vi "delay chart.vi"(8 "Spec":dbl, 9 "Des.":string="TDD11", 10 "Impedance Data":dbl[](array[numeric]), 11 "Time Array":dbl[](array[numeric])) -> (0 "Test Summary":string, 1 "test passed?":bool=TRUE caption="Test Pass?", 2 "Test Data":T2, 3 "Impedance Chart":T1(graph), 5 "delay":dbl)   [LabVIEW 2011]
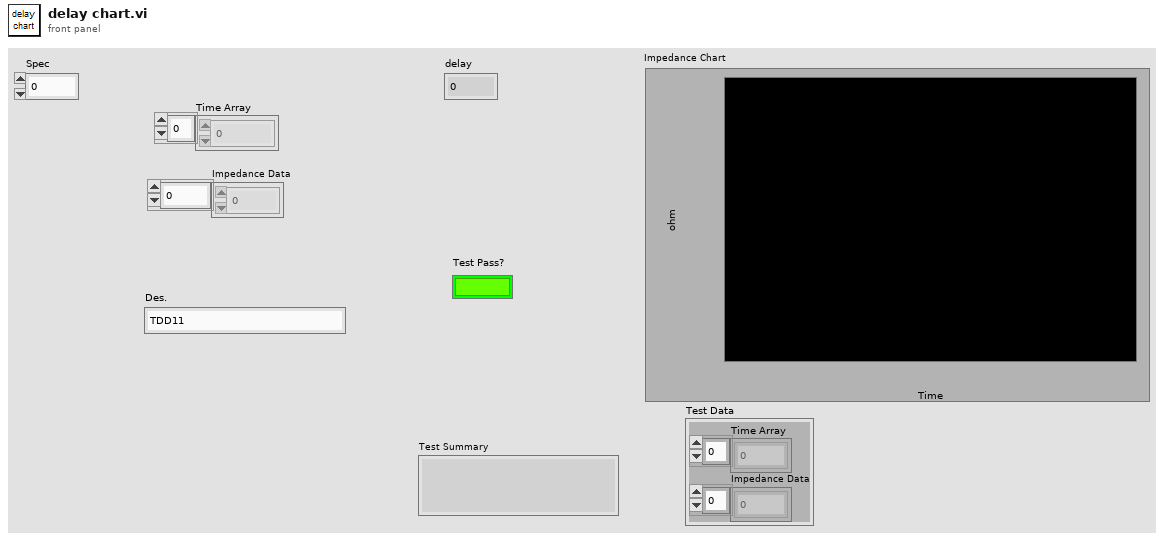
[diagram p1: front panel]
types:
  T1 = cluster{"Time Array":dbl[], "Lower Spec":dbl[]}[]
  T2 = cluster{"Time Array":dbl[], "Impedance Data":dbl[]}
  T3 = cluster{"Time Array":dbl[], "Impedance Data":dbl[]}[]
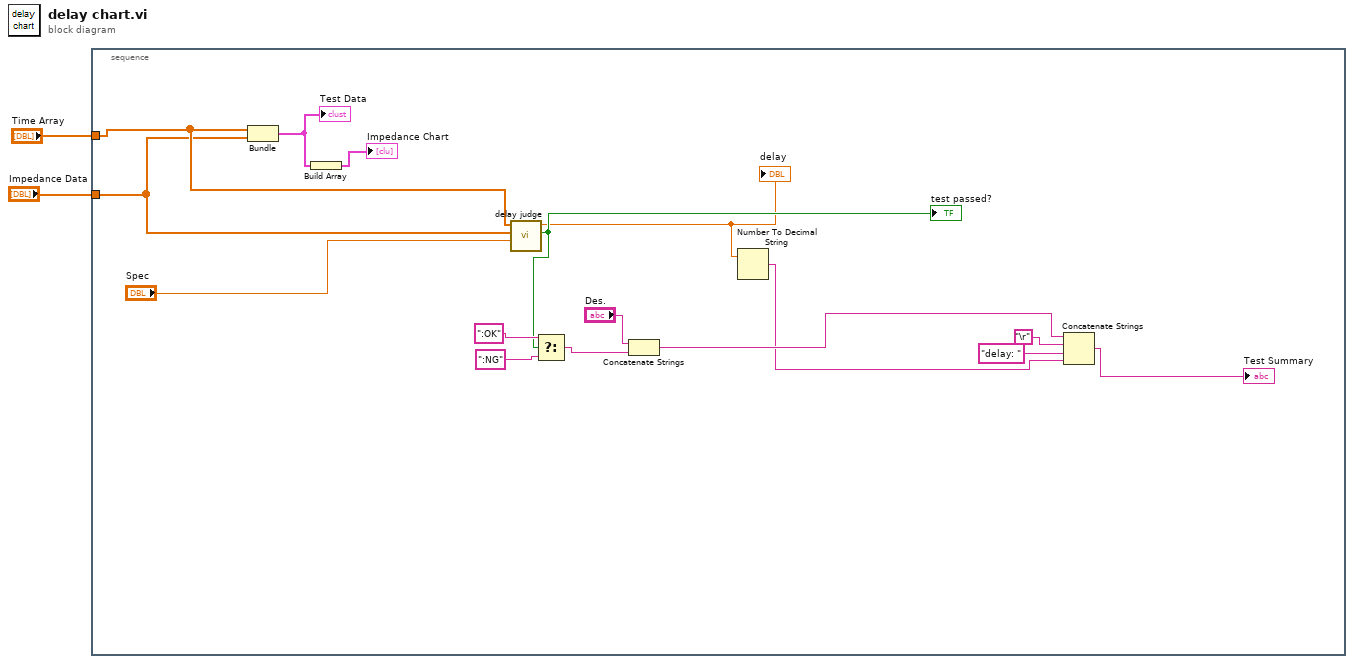
[diagram p0: block diagram]
diagram:
  n1 = stacked-sequence {
    tunnel: "Time Array" -> [w8]
    tunnel: "Impedance Data" -> [w7]
    frame #0 {
      n2 = Bundle("Time Array"=w8, "Impedance Data"=w7) -> (w9:T2)  [unwired: 1 in]
      "Test Data" <- w9
      n3 = Build Array(w9) -> (→"Impedance Chart":T3)
      n4 = call "delay judge.vi"("Spec"="Spec", "Impedance Data"=w7, "Time Array"=w8) -> ("result"=w6:bool, "delay"=w5:dbl)  [unwired: 7 in]
      "test passed?" <- w6
      "delay" <- w5
      n5 = Select(t=":OK" ("Des."), s=w6, f=":NG" ("Des.")) -> (s? t:f=w12:string)
      n6 = Concatenate Strings("Des.", w12) -> (w10:string)
      n7 = Number To Decimal String(number=w5) -> (decimal integer string=w4:string)  [unwired: 1 in]
      n8 = Concatenate Strings(w10, "\r", "delay: " ("字符串"), w4) -> (→"Test Summary":string)
    }
  }
